vi "LCR_ReadAll.vi"(8 "error in (no error)":errorcluster, 9 "Data_In":T1, 10 "Configuration Cluster":T3={"General"={"Config.ini"=path "", "Default Logging Path"=path ""}, "Hardware"={"AHC VISA COM"="", "Measure Rate (1/s)"=0, "Global T VAR"="", "Global B VAR"=""}, "Operation"={"Operation Mode"=enum."Idle-Off", "Status"="", "NewLog?"=FALSE}}) -> (0 "error out":errorcluster, 1 "Data_Out":T1, 2 "Configuration Cluster 2":T3={"General"={"Config.ini"=path "", "Default Logging Path"=path ""}, "Hardware"={"AHC VISA COM"="", "Measure Rate (1/s)"=0, "Global T VAR"="", "Global B VAR"=""}, "Operation"={"Operation Mode"=enum."Idle-Off", "Status"="", "NewLog?"=FALSE}}, 4 "Secondary Measurement":dbl, 6 "Primary Measurement":dbl)   [LabVIEW 2021]
uses:
  Config_Cluster.ctl
  Mode_Enum.ctl
  Data_Cluster.ctl
  Measurement_Cluster.ctl
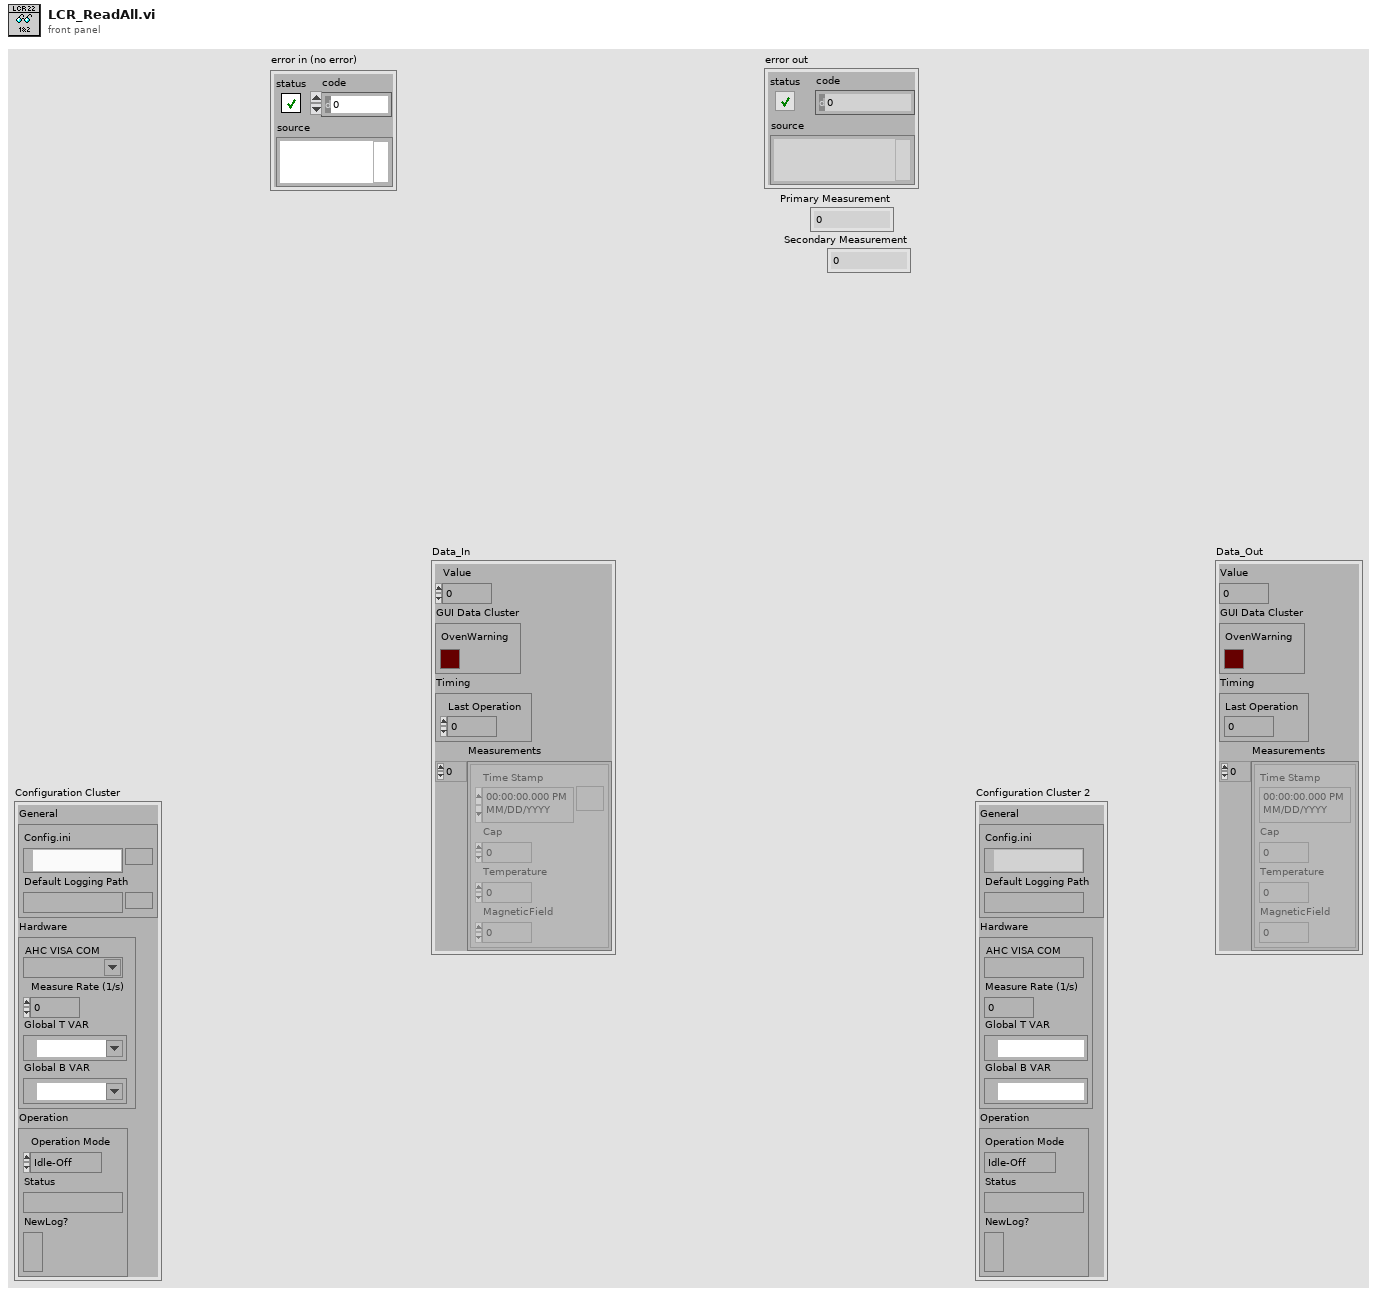
[diagram p1: front panel]
types:
  T1 = typedef "Data_Cluster.ctl" = cluster{"Value":dbl, "GUI Data Cluster":cluster{"OvenWarning":bool}, "Timing":cluster{"Last Operation":dbl}, "Measurements":T2[]}
  T2 = typedef "Measurement_Cluster.ctl" = cluster{"Time Stamp":timestamp, "Cap":dbl, "Temperature":dbl, "MagneticField":dbl}
  T3 = typedef "Config_Cluster.ctl" = cluster{"General":cluster{"Config.ini":path, "Default Logging Path":path}, "Hardware":cluster{"AHC VISA COM":refnum<visa-resource-name>, "Measure Rate (1/s)":i32, "Global T VAR":refnum<k21>, "Global B VAR":refnum<k21>}, "Operation":cluster{"Operation Mode":T4, "Status":string, "NewLog?":bool}}
  T4 = typedef "Mode_Enum.ctl" = enum16{"Logging", "Idle-Off", "Idle"}
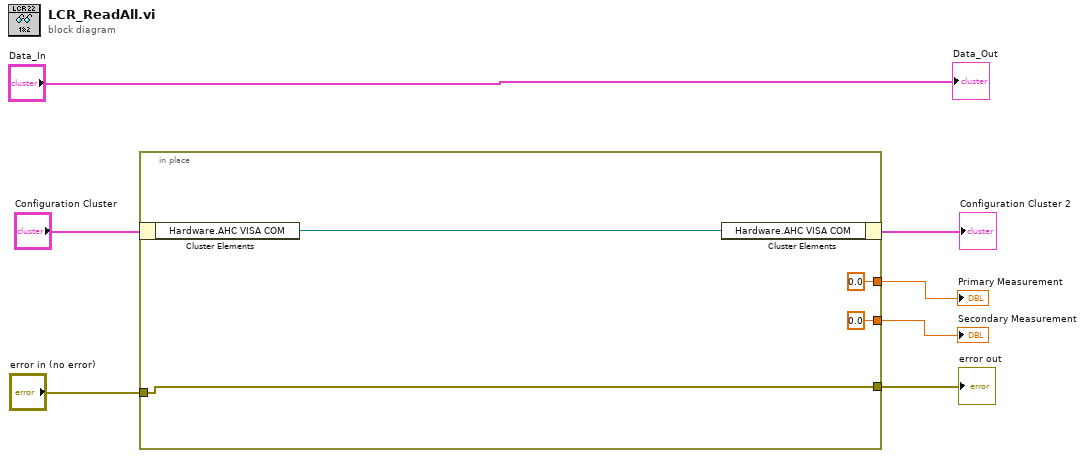
[diagram p0: block diagram]
diagram:
  n1 = in-place {
    in-place-border: "error in (no error)" -> [w10]
    in-place-border: [w10] -> w5
    in-place-border: [0.0 ("Primary Measurement")] -> w4
    in-place-border: [0.0 ("Secondary Measurement")] -> w3
    n2 = in-place-cluster #1("Configuration Cluster") -> ("Hardware.AHC VISA COM"=w11:refnum<visa-resource-name>)
    n3 = in-place-cluster #1("Hardware.AHC VISA COM"=w11) -> (→"Configuration Cluster 2":T3)
  }
  "error out" <- w5
  "Primary Measurement" <- w4
  "Secondary Measurement" <- w3
  "Data_Out" <- "Data_In"
